vi "Create UEGO.vi"(8 "error in (no error)":errorcluster, 11 "Parent Ref in":T1 format="%.0x") -> (0 "error out":errorcluster, 3 "Parent Ref out":T1 format="%.0x")   [LabVIEW 2015, in "DCM System Explorer.lvlib"]
uses:
  DCM System Explorer.lvlib
  <vilib>/NI Veristand/Custom Device API/Custom Device Item Ref.ctl
  <vilib>/NI Veristand/Custom Device API/Custom Device Channel Type.ctl
  Shared/DCM Constants and GUIDs.vi
  <vilib>/NI VeriStand/Custom Device API/Custom Device API.lvlib
  DCM Shared.lvlib
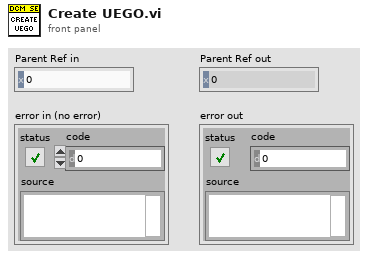
[diagram p1: front panel]
types:
  T1 = typedef "Custom Device API.lvlib/Custom Device Item Ref.ctl" = u64
  T2 = typedef "Custom Device API.lvlib/Custom Device Channel Type.ctl" = enum16{"Input", "Output"}
  T3 = typedef "DCM Shared.lvlib/Channel.ctl" = cluster{"Name":string, "Units":string, "Default":dbl, "Description":string}
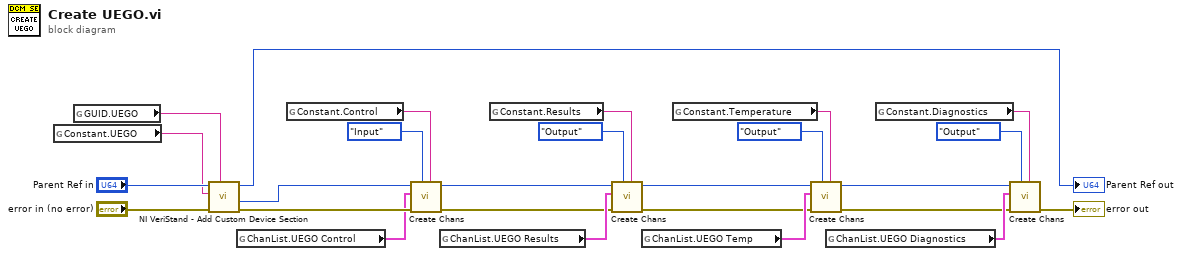
[diagram p0: block diagram]
diagram:
  n1 = global read "DCM Constants and GUIDs.vi" "Constant.UEGO"() -> (w24:string)
  n2 = global read "DCM Constants and GUIDs.vi" "GUID.UEGO"() -> (w23:string)
  n3 = call <vilib>:"NI VeriStand - Add Custom Device Section.vi"("GUID (Default Section)"=w23, "error in (no error)"="error in (no error)", "Section Name"=w24, "Parent Ref in"="Parent Ref in") -> ("error out"=w19:errorcluster, "Section Ptr"=w21:T1, "Parent Ref out"=→"Parent Ref out":T1)  [unwired: 4 in, 1 out]
  n4 = global read "DCM Constants and GUIDs.vi" "ChanList.UEGO Control"() -> (w18:T3[])
  n5 = global read "DCM Constants and GUIDs.vi" "Constant.Control"() -> (w20:string)
  n6 = call "Create Chans.vi"("New Section Name (none)"=w20, "Type"=Custom_Device_Channel_Type."Input", "error in (no error)"=w19, "Channels"=w18, "Section Ptr"=w21) -> ("error out"=w7:errorcluster, "Section Ptr dup"=w8:T1)  [unwired: 3 in, 2 out]
  n7 = global read "DCM Constants and GUIDs.vi" "ChanList.UEGO Results"() -> (w16:T3[])
  n8 = global read "DCM Constants and GUIDs.vi" "Constant.Results"() -> (w15:string)
  n9 = call "Create Chans.vi"("New Section Name (none)"=w15, "Type"=Custom_Device_Channel_Type."Output", "error in (no error)"=w7, "Channels"=w16, "Section Ptr"=w8) -> ("error out"=w9:errorcluster, "Section Ptr dup"=w10:T1)  [unwired: 3 in, 2 out]
  n10 = global read "DCM Constants and GUIDs.vi" "ChanList.UEGO Temp"() -> (w11:T3[])
  n11 = global read "DCM Constants and GUIDs.vi" "Constant.Temperature"() -> (w12:string)
  n12 = call "Create Chans.vi"("New Section Name (none)"=w12, "Type"=Custom_Device_Channel_Type."Output", "error in (no error)"=w9, "Channels"=w11, "Section Ptr"=w10) -> ("error out"=w2:errorcluster, "Section Ptr dup"=w3:T1)  [unwired: 3 in, 2 out]
  n13 = global read "DCM Constants and GUIDs.vi" "ChanList.UEGO Diagnostics"() -> (w6:T3[])
  n14 = global read "DCM Constants and GUIDs.vi" "Constant.Diagnostics"() -> (w5:string)
  n15 = call "Create Chans.vi"("New Section Name (none)"=w5, "Type"=Custom_Device_Channel_Type."Output", "error in (no error)"=w2, "Channels"=w6, "Section Ptr"=w3) -> ("error out"=→"error out":errorcluster)  [unwired: 3 in, 3 out]
